vi "Set Input Impedance and Max Freq for Channel(s).vi"(7 "Channel(s)":T1[](array[typedef]), 8 "error in (no error)":errorcluster, 11 "PXIe5105 in":refnum<class "PXIe5105.lvclass">) -> (0 "error out":errorcluster, 3 "PXIe5105 out":refnum<class "PXIe5105.lvclass">)   [LabVIEW 2018, in "PXIe5105.lvlib" / "PXIe5105.lvclass"]
uses:
  PXIe5105.lvclass
  PPLs/Oscilloscope/Parent/Oscilloscope.lvlibp/Custom Controls/Analog Channels.ctl
  PXIe5105.lvclass/PXIe5105.ctl
  PPLs/Oscilloscope/Parent/Oscilloscope.lvlibp
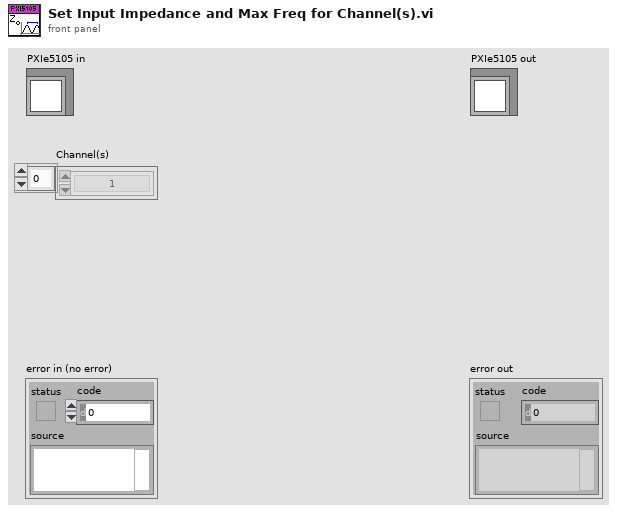
[diagram p1: front panel]
types:
  T1 = typedef "Oscilloscope.lvlibp/Analog Channels.ctl" = enum16{"1", "2", "3", "4", "5", "6", "7", "8", "9", "10", "11", "12", "13", "14", "15", "16"}
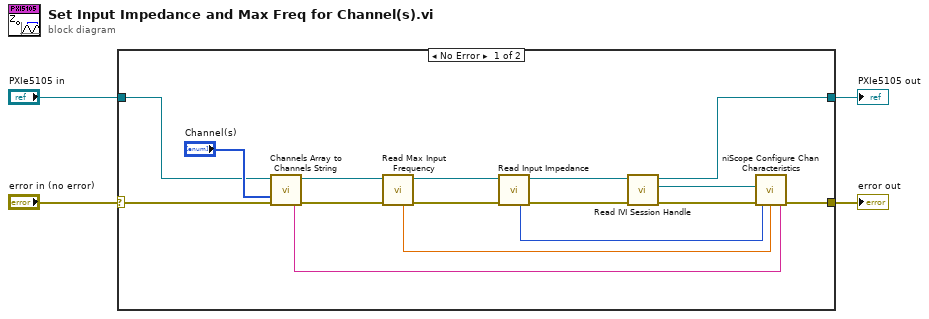
[diagram p0: block diagram]
diagram:
  n1 = case shown="No Error" "error in (no error)" {
    selector: "error in (no error)" -> [w7 w22]
    tunnel: [w19 w22] -> w3
    tunnel: [w9 w21] -> w1
    tunnel: "PXIe5105 in" -> [w8 w21]
    frame No Error {
      n2 = call "Channels Array to Channels String.vi"("error in (no error)"=w7, "Channel(s) Array"="Channel(s)", "PXIe5105 in"=w8) -> ("error out"=w14:errorcluster, "Channels String"=w18:string, "PXIe5105 out"=w15:refnum<class "PXIe5105.lvclass">)  [unwired: 6 in]
      n3 = call "Read Max Input Frequency.vi"("error in (no error)"=w14, "PXIe5105 in"=w15) -> ("error out"=w12:errorcluster, "Max Input Frequency"=w16:dbl, "PXIe5105 out"=w13:refnum<class "PXIe5105.lvclass">)  [unwired: 7 in]
      n4 = call "Read Input Impedance.vi"("error in (no error)"=w12, "PXIe5105 in"=w13) -> ("error out"=w10:errorcluster, "Input Impedance"=w17:u32, "PXIe5105 out"=w11:refnum<class "PXIe5105.lvclass">)  [unwired: 7 in]
      n5 = call "Read IVI Session Handle.vi"("error in (no error)"=w10, "PXIe5105 in"=w11) -> ("error out"=w5:errorcluster, "IVI Session Handle"=w6:refnum<k15>, "PXIe5105 out"=w9:refnum<class "PXIe5105.lvclass">)  [unwired: 7 in]
      n6 = call <instrlib>:"niScope Configure Chan Characteristics.vi"("instrument handle"=w6, "channels"=w18, "input impedance"=w17, "maximum input frequency"=w16, "error in"=w5) -> ("error out"=w19:errorcluster)  [unwired: 9 in, 1 out]
    }
    frame Error {
    }
  }
  "error out" <- w3
  "PXIe5105 out" <- w1
